vi "Zustandsautomat_CG-Check.vi"(6 "Zustand":T1, 8 "Fehler 2":bool, 9 "Span Eingang":string, 10 "Index":i32, 11 "Istwerte":dbl[](array[numeric])) -> (0 "Fehler":bool, 1 "Anzeige":string, 2 "Zeitanzeige":string, 3 "Verstrichene Zeit":sgl, 4 "Zustand":T1)   [LabVIEW 2020, in "Erweiterte Konfig.lvlib" / "CG-Check Konfig.lvlib"]
uses:
  CG-Check Konfig.lvlib
  Zustand CG-Check.ctl
  Aktion_CG-Check.ctl
  Sprachverwaltung/FGV Aktion Tabelle zerlegen.ctl
  Stoerungen/Stoerungen Messgeraet/Aktionen Kommunikation Stoerung.ctl
  Aktion_CG-Check_Protokoll.ctl
  FT-IR/FT-IR.lvlib
  Stoerungen/Stoerungen.lvlib
  Sprachverwaltung/Sprachverwaltung.lvlib
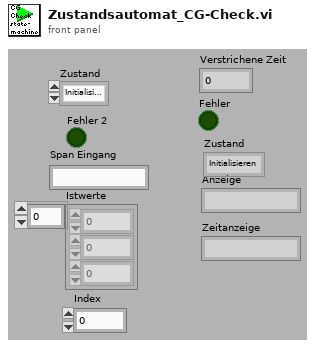
[diagram p1: front panel]
types:
  T1 = typedef "Erweiterte Konfig.lvlib/CG-Check Konfig.lvlib/Zustand CG-Check.ctl" = enum16{"Initialisieren", "Aufschaltdauer", "Prüfdauer", "Auswertung", "Fertig"}
  T2 = typedef "Sprachverwaltung.lvlib/FGV Aktion Tabelle zerlegen.ctl" = enum16{"laden", "vereinzeln", "speichern"}
  T3 = typedef "Erweiterte Konfig.lvlib/CG-Check Konfig.lvlib/Aktion_CG-Check.ctl" = enum16{"lesen", "schreiben", "laden", "Komponente", "Aktive?", "speichern"}
  T4 = typedef "Stoerungen.lvlib/Aktionen Kommunikation Stoerung.ctl" = enum16{"lesen", "init", "FT-IR Komm", "FT-IR Betriebsart", "FT-IR Hintergrund", "cRIO Komm", "PNS Komm", "Dichtheitstest", "Life Bit", "FTIR Komm AK", "PMA Komm", "FID Komm", "PMA Cal", "FID Ch4 Cal", "FID THC Cal", "Cal Timeout", "VFS 1 Komm", "VFS 2 Komm", "VFS 3 Komm", "VFS 4 Komm", "TRE 08 Komm", "CG-Test vorzeitig", "CG-Test Span 1", "CG-Test Span 2", "CG-Test Span 3", "CG-Test Messgas", "CG-Test löschen", "Test", "Amium AK", "AK Recept konfig", "AK Name konfig", "AK EKFG konfig"}
  T5 = typedef "Erweiterte Konfig.lvlib/CG-Check Konfig.lvlib/Aktion_CG-Check_Protokoll.ctl" = enum16{"Zeitstempel", "Sollwerte", "Istwerte", "Vorzeitig beendet", "Auswerten", "Speichern", "Lesen"}
  T6 = cluster{"Aufschaltdauer":sgl, "Prüfdauer":sgl, "Mittelwertanzahl":u8}
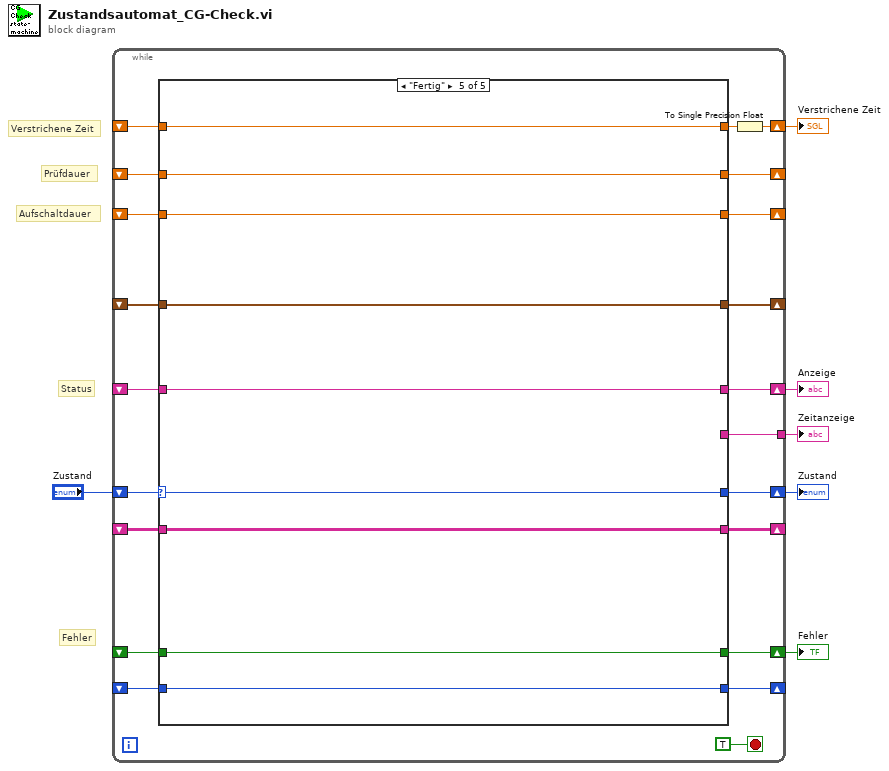
[diagram p0: block diagram]
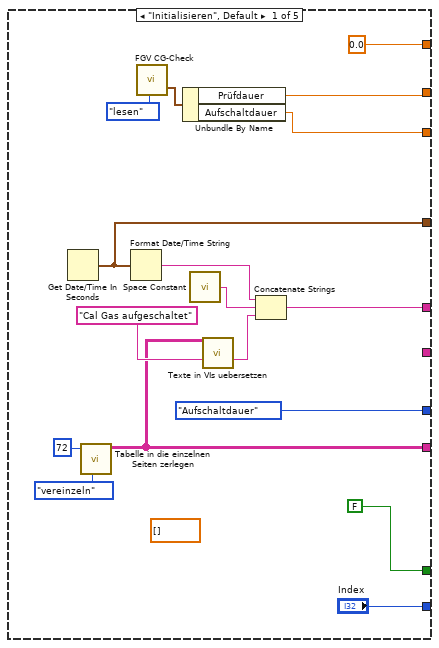
[diagram p2: hidden frame]
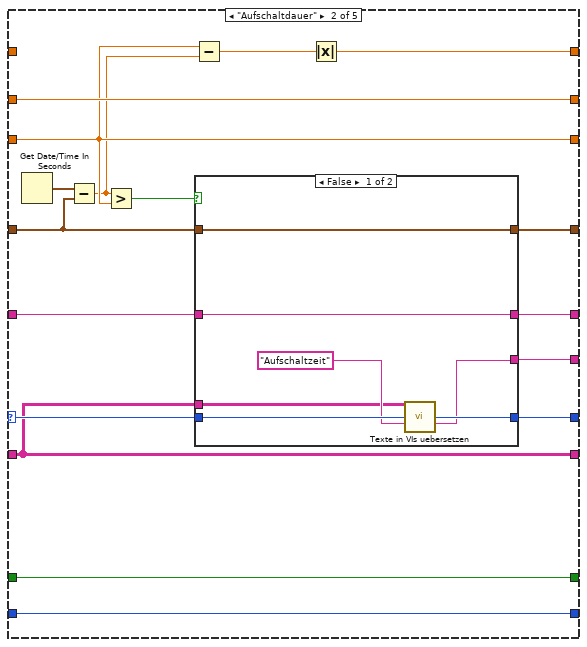
[diagram p3: hidden frame]
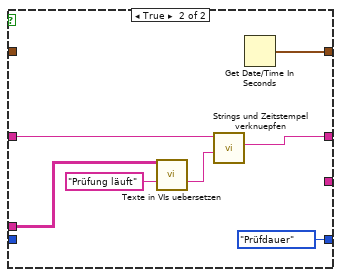
[diagram p4: hidden frame]
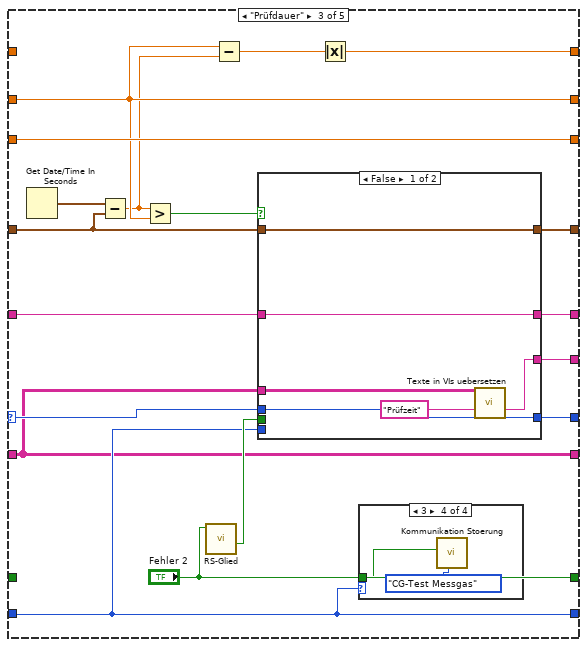
[diagram p5: hidden frame]
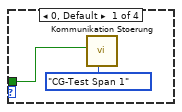
[diagram p6: hidden frame]
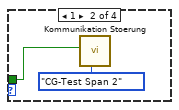
[diagram p7: hidden frame]
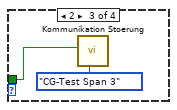
[diagram p8: hidden frame]
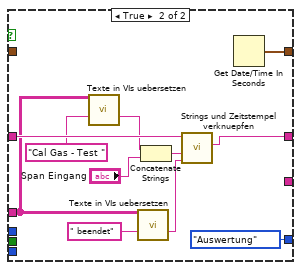
[diagram p9: hidden frame]
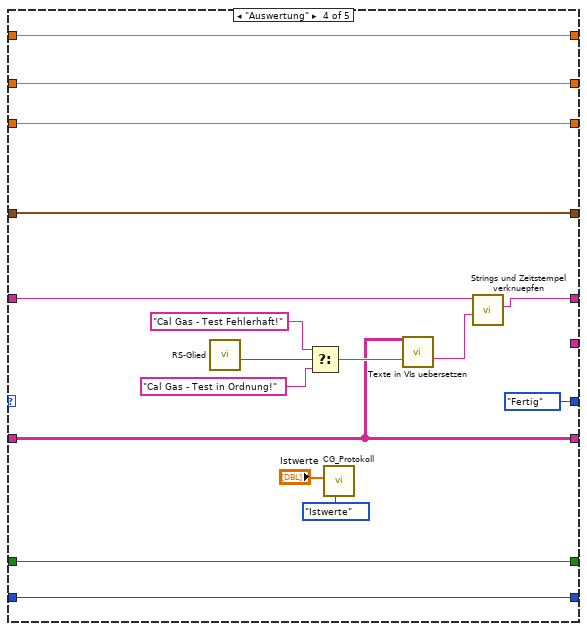
[diagram p10: hidden frame]
diagram:
  # "Fehler"
  # "Verstrichene Zeit"
  # "Status"
  # "Prüfdauer"
  # "Aufschaltdauer"
  n1 = while {
    shift-right: [w26] -> w5
    shift-left: _ -> [w17]
    shift-right: [w24] -> _
    shift-left: _ -> [w18]
    shift-right: [w25] -> _
    shift-left: _ -> [w19]
    shift-right: [w13] -> w6
    shift-left: _ -> [w20]
    shift-right: [w21] -> w2
    shift-left: _ -> [w16]
    shift-right: [w15] -> _
    shift-left: _ -> [w14]
    shift-right: [w23] -> w3
    shift-left: "Zustand" -> [w12]
    tunnel: [w11] -> w1
    shift-right: [w10] -> _
    shift-left: _ -> [w9]
    shift-right: [w7] -> _
    shift-left: _ -> [w8]
    stop <- TRUE stop-if-true
    n2 = case shown="\"Fertig\"" w12 {
      selector: w12 -> [_ w56 w85 _ w138]
      tunnel: [w42 w55 w87 w133 w139] -> w26
      tunnel: [w34 w51 w88 w132 w141] -> w25
      tunnel: [w35 w53 w84 w131 w142] -> w24
      tunnel: [Zustand_CG-Check."Aufschaltdauer" ("Zustand") w57 w86 Zustand_CG-Check."Fertig" ("Zustand") w138] -> w23
      tunnel: [0.0 w47 w80 w130 w143] -> w22
      tunnel: [FALSE w52 "Fehler 2" w122 w137] -> w21
      tunnel: w20 -> [_ _ _ w130 w143]
      tunnel: w19 -> [_ w51 w88 w132 w141]
      tunnel: w18 -> [_ w53 w84 w131 w142]
      tunnel: w17 -> [_ w54 w77 w134 w139]
      tunnel: w16 -> [_ w52 _ w122 w137]
      tunnel: [w37 w59 w90 w128 w140] -> w15
      tunnel: w14 -> [_ w60 w91 w128 w140]
      tunnel: [_ w49 w81 _ _] -> w11
      tunnel: ["Index" w46 w76 w121 w136] -> w10
      tunnel: w9 -> [_ w46 w76 w121 w136]
      tunnel: w8 -> [_ w45 w75 w118 w135]
      tunnel: [w28 w45 w75 w118 w135] -> w7
      frame "Initialisieren", Default {
        (unwired) dbl[] []
        n3 = Get Date/Time In Seconds() -> (seconds since 1Jan1904=w37:timestamp)
        n4 = call "Tabelle in die einzelnen Seiten zerlegen.vi"("Aktion"=FGV_Aktion_Tabelle_zerlegen."vereinzeln", "Index (Seite)"=72) -> ("Sprachliste"=w28:string[][])  [unwired: 7 in, 2 out]
        n5 = Format Date/Time String(seconds (now)=w37) -> (date/time string=w44:string)  [unwired: 2 in]
        n6 = call "FGV CG-Check.vi"("Aktion"=Aktion_CG-Check."lesen") -> ("Cluster"=w36:T6)  [unwired: 11 in, 7 out]
        n7 = Unbundle By Name(w36) -> ("Prüfdauer"=w35:sgl, "Aufschaltdauer"=w34:sgl)
        n8 = call <vilib>:"Space Constant.vi"() -> ("String"=w43:string)
        n9 = call "Texte in VIs uebersetzen.vi"("Sprachliste"=w28, "String zum Übersetzen"="Cal Gas aufgeschaltet" ("String")) -> ("String zum Übersetzen"=w31:string)  [unwired: 9 in, 4 out]
        n10 = Concatenate Strings(w44, w43, w31) -> (w42:string)
      }
      frame "Aufschaltdauer" {
        n11 = Get Date/Time In Seconds() -> (seconds since 1Jan1904=w61:timestamp)
        n12 = Subtract(x=w61, y=w60) -> (x-y=w50:dbl)
        n13 = Greater?(x=w50, y=w51) -> (0:w58:bool)
        n14 = Subtract(x=w51, y=w50) -> (x-y=w48:dbl)
        n15 = case shown="False" w58 {
          tunnel: w60 -> [w67 _]
          tunnel: [w67 w74] -> w59
          tunnel: [w66 Zustand_CG-Check."Prüfdauer" ("Zustand")] -> w57
          tunnel: w56 -> [w66 _]
          tunnel: [w65 w73] -> w55
          tunnel: w54 -> [w65 w72]
          tunnel: [w63 _] -> w49
          tunnel: w45 -> [w62 w68]
          frame False {
            n16 = call "Texte in VIs uebersetzen.vi"("Sprachliste"=w62, "String zum Übersetzen"="Aufschaltzeit") -> ("String zum Übersetzen"=w63:string)  [unwired: 9 in, 4 out]
          }
          frame True {
            n17 = call "Texte in VIs uebersetzen.vi"("Sprachliste"=w68, "String zum Übersetzen"="Prüfung läuft" ("Eingagns String")) -> ("String zum Übersetzen"=w69:string)  [unwired: 9 in, 4 out]
            n18 = call "Strings und Zeitstempel verknuepfen.vi"("String 1 hinzufügen"=w69, "Eingagns String"=w72) -> ("Verknüpfter String"=w73:string)  [unwired: 9 in]
            n19 = Get Date/Time In Seconds() -> (seconds since 1Jan1904=w74:timestamp)
          }
        }
        n20 = Absolute Value(x=w48) -> (abs(x)=w47:dbl)
      }
      frame "Prüfdauer" {
        n21 = Get Date/Time In Seconds() -> (seconds since 1Jan1904=w92:timestamp)
        n22 = Subtract(x=w92, y=w91) -> (x-y=w83:dbl)
        n23 = Greater?(x=w83, y=w84) -> (0:w89:bool)
        n24 = call "RS-Glied.vi"("set"="Fehler 2") -> ("Fehler"=w78:bool)  [unwired: 10 in]
        n25 = Subtract(x=w84, y=w83) -> (x-y=w82:dbl)
        n26 = case shown="False" w89 {
          tunnel: w91 -> [w106 _]
          tunnel: [w106 w117] -> w90
          tunnel: w77 -> [w104 w116]
          tunnel: [w104 w115] -> w87
          tunnel: [w105 Zustand_CG-Check."Auswertung" ("Zustand")] -> w86
          tunnel: w85 -> [w105 _]
          tunnel: [w102 _] -> w81
          tunnel: w76 -> [_ _]
          tunnel: w78 -> [_ _]
          tunnel: w75 -> [w101 w107]
          frame False {
            n27 = call "Texte in VIs uebersetzen.vi"("Sprachliste"=w101, "String zum Übersetzen"="Prüfzeit") -> ("String zum Übersetzen"=w102:string)  [unwired: 9 in, 4 out]
          }
          frame True {
            n28 = call "Texte in VIs uebersetzen.vi"("Sprachliste"=w107, "String zum Übersetzen"="Cal Gas - Test " ("String 1 hinzufügen")) -> ("String zum Übersetzen"=w108:string)  [unwired: 9 in, 4 out]
            n29 = call "Texte in VIs uebersetzen.vi"("Sprachliste"=w107, "String zum Übersetzen"=" beendet") -> ("String zum Übersetzen"=w110:string)  [unwired: 9 in, 4 out]
            n30 = Concatenate Strings(w108, "Span Eingang") -> (w113:string)
            n31 = call "Strings und Zeitstempel verknuepfen.vi"("String 2 hinzufügen"=w110, "String 1 hinzufügen"=w113, "Eingagns String"=w116) -> ("Verknüpfter String"=w115:string)  [unwired: 8 in]
            n32 = Get Date/Time In Seconds() -> (seconds since 1Jan1904=w117:timestamp)
          }
        }
        n33 = Absolute Value(x=w82) -> (abs(x)=w80:dbl)
        n34 = case shown="3" w76 {
          tunnel: "Fehler 2" -> [w93 w95 w97 w99]
          frame 0, Default {
            n35 = call "Kommunikation Stoerung.vi"("Aktionen"=Aktionen_Kommunikation_Stoerung."CG-Test Span 1", "ERROR"=w93) -> ()  [unwired: 9 in, 1 out]
          }
          frame 1 {
            n36 = call "Kommunikation Stoerung.vi"("Aktionen"=Aktionen_Kommunikation_Stoerung."CG-Test Span 2", "ERROR"=w95) -> ()  [unwired: 9 in, 1 out]
          }
          frame 2 {
            n37 = call "Kommunikation Stoerung.vi"("Aktionen"=Aktionen_Kommunikation_Stoerung."CG-Test Span 3", "ERROR"=w97) -> ()  [unwired: 9 in, 1 out]
          }
          frame 3 {
            n38 = call "Kommunikation Stoerung.vi"("Aktionen"=Aktionen_Kommunikation_Stoerung."CG-Test Messgas", "ERROR"=w99) -> ()  [unwired: 9 in, 1 out]
          }
        }
      }
      frame "Auswertung" {
        n39 = call "RS-Glied.vi"() -> ("Fehler"=w127:bool)  [unwired: 11 in]
        n40 = Select(t="Cal Gas - Test Fehlerhaft!", s=w127, f="Cal Gas - Test in Ordnung!") -> (s? t:f=w120:string)
        n41 = call "CG_Protokoll.vi"("Aktion"=Aktion_CG-Check_Protokoll."Istwerte", "Istwerte"="Istwerte") -> ()  [unwired: 8 in, 2 out]
        n42 = call "Texte in VIs uebersetzen.vi"("Sprachliste"=w118, "String zum Übersetzen"=w120) -> ("String zum Übersetzen"=w119:string)  [unwired: 9 in, 4 out]
        n43 = call "Strings und Zeitstempel verknuepfen.vi"("String 1 hinzufügen"=w119, "Eingagns String"=w134) -> ("Verknüpfter String"=w133:string)  [unwired: 9 in]
      }
      frame "Fertig" {
      }
    }
    n44 = To Single Precision Float(number=w22) -> (single precision float=w13:sgl)
  }
  "Verstrichene Zeit" <- w6
  "Anzeige" <- w5
  "Zustand" <- w3
  "Fehler" <- w2
  "Zeitanzeige" <- w1
